vi "AVS_SetAnalogOut.vi"(0 "a_hDevice":i32, 7 "a_PortId":u8, 11 "a_Value":sgl) -> (4 "Output Value":i32)   [LabVIEW 2009]
uses:
  avaspecx64.dll
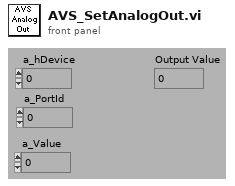
[diagram p1: front panel]
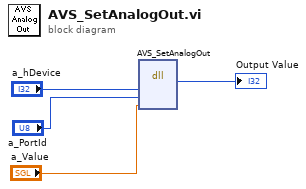
[diagram p0: block diagram]
diagram:
  n1 = dll-call lib="E:/Documents and Settings/mattc/Libraries/Avaspec_Library/trunk/demo_64bit/LabView/LabViewSingleChan/avaspecx64.dll" fn="AVS_SetAnalogOut"("a_hDevice"="a_hDevice", "a_PortId"="a_PortId", "a_Value"="a_Value") -> ("return type"=→"Output Value":i32)  [unwired: 6 in, 2 out]
